vi "Create Logs Queue.vi"(8 "Error In":errorcluster, 11 "EventLog in":refnum<class "ErrorLog.lvclass">) -> (0 "Error Out":errorcluster, 3 "EventLog out":refnum<class "ErrorLog.lvclass">)   [LabVIEW 2019, in "ErrorLog.lvlib" / "ErrorLog.lvclass"]
uses:
  ErrorLog.lvclass
  Classes/Error/Error.lvclass
  ErrorLog.lvclass/ErrorLog.ctl
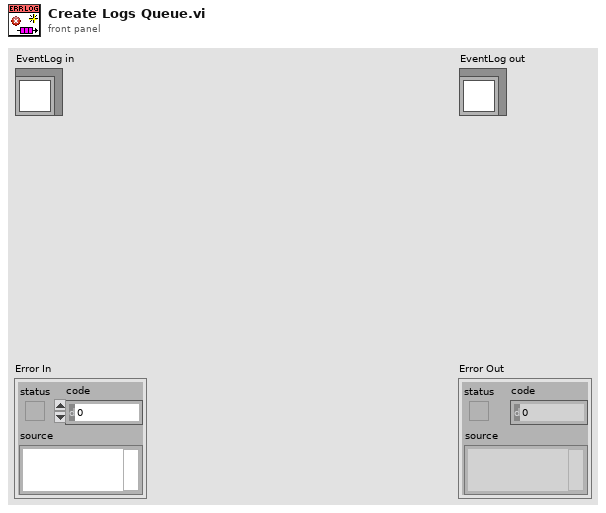
[diagram p1: front panel]
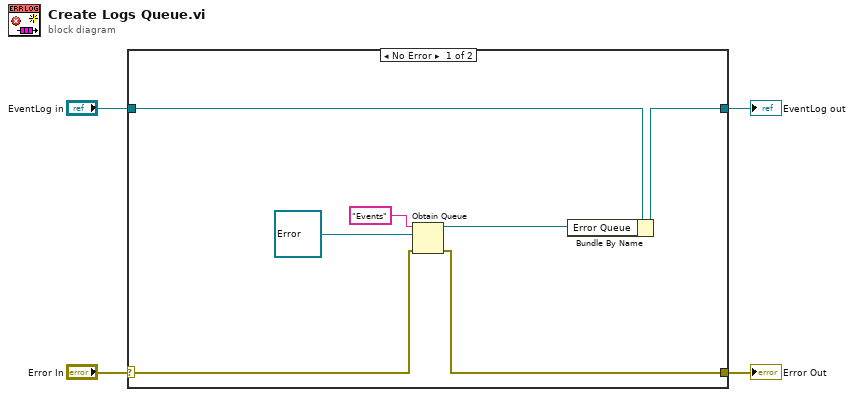
[diagram p0: block diagram]
diagram:
  n1 = case shown="No Error" "Error In" {
    selector: "Error In" -> [w8 w13]
    tunnel: [w7 w13] -> w4
    tunnel: [w6 w12] -> w3
    tunnel: "EventLog in" -> [w11 w12]
    frame No Error {
      n2 = Obtain Queue(name (unnamed)="Events", element data type=refnum<class "Error.lvclass"> refnum ("Events.lvclass"), error in (no error)=w8) -> (queue out=w5:refnum<queue>, error out=w7:errorcluster)  [unwired: 2 in, 1 out]
      n3 = Bundle By Name(cluster=w11, "Error Queue"=w5) -> (w6:refnum<class "ErrorLog.lvclass">)
    }
    frame Error {
    }
  }
  "Error Out" <- w4
  "EventLog out" <- w3
